vi "Init.vi"(8 "error in (no error)":errorcluster, 10 "Channel":i16, 11 "TrialBasedExperiment in":refnum<class "WNOriDiscExperiment.lvclass">) -> (0 "error out":errorcluster, 3 "TrialBasedExperiment out":refnum<class "WNOriDiscExperiment.lvclass">)   [LabVIEW 2014, in "WNOriDiscExperiment.lvclass"]
uses:
  WNOriDiscExperiment.lvclass
  TwoAfcEye/TwoAfcEye.lvclass
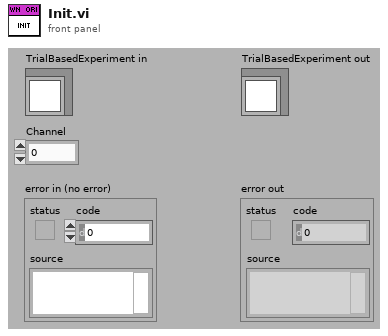
[diagram p1: front panel]
types:
  T1 = cluster{"Intertrial":dbl, "AcquireFixation":dbl, "HoldFixation":dbl, "DelayPeriod":dbl, "ResponsePeriod":dbl}
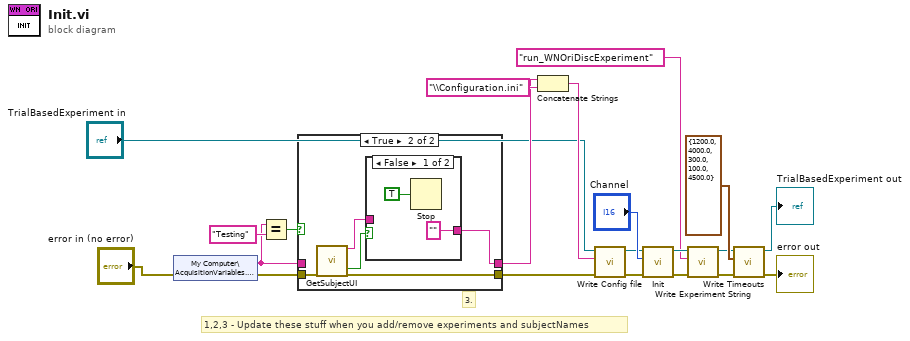
[diagram p0: block diagram]
diagram:
  # "1,2,3 - Update these stuff when you add/remove experiments and subjectNames"
  # "3."
  n1 = shared-variable "My Computer\\AcquisitionVariables.lvlib\\Subject"(error in="error in (no error)") -> (w17:string, error out=w16:errorcluster)
  n2 = Equal?(x=w17, y="Testing") -> (x = y?=w19:bool)
  n3 = case shown="True" w19 {
    tunnel: [w23 w28] -> w14
    tunnel: w17 -> [w23 _]
    tunnel: w16 -> [w22 w24]
    tunnel: [w22 w25] -> w15
    frame False {
    }
    frame True {
      n4 = call "GetSubjectUI.vi"("error in (no error)"=w24) -> ("subjectSelected"=w27:string, "OK"=w26:bool, "error out"=w25:errorcluster)  [unwired: 16 in]
      n5 = case shown="False" w26 {
        tunnel: w27 -> [_ w31]
        tunnel: ["" ("subjectSelected") w31] -> w28
        frame False {
          n6 = Stop(stop? (T)=TRUE) -> ()
        }
        frame True {
        }
      }
    }
  }
  n7 = Concatenate Strings(w14, "\\Configuration.ini") -> (w21:string)
  n8 = call-dynamic "Write Config file.vi"("error in (no error)"=w15, "Config file"=w21, "TrialBasedExperiment in"="TrialBasedExperiment in") -> ("error out"=w5:errorcluster, "TrialBasedExperiment out"=w6:refnum<class "WNOriDiscExperiment.lvclass">)  [unwired: 7 in]
  n9 = call-parent "Init.vi"("error in (no error)"=w5, "Channel"="Channel", "TrialBasedExperiment in"=w6) -> ("error out"=w4:errorcluster, "TrialBasedExperiment out"=w7:refnum<class "WNOriDiscExperiment.lvclass">)  [unwired: 7 in]
  n10 = call-dynamic "Write Experiment String.vi"("error in (no error)"=w4, "Experiment String"="run_WNOriDiscExperiment" ("string"), "TrialBasedExperiment in"=w7) -> ("error out"=w10:errorcluster, "TrialBasedExperiment out"=w9:refnum<class "WNOriDiscExperiment.lvclass">)  [unwired: 7 in]
  n11 = call-dynamic "Write Timeouts.vi"("error in (no error)"=w10, "Timeouts"=T1 {"Intertrial"=1200.0, "AcquireFixation"=4000.0, "HoldFixation"=300.0, "DelayPeriod"=100.0, "ResponsePeriod"=4500.0}, "TrialBasedExperiment in"=w9) -> ("error out"=→"error out":errorcluster, "TrialBasedExperiment out"=→"TrialBasedExperiment out":refnum<class "WNOriDiscExperiment.lvclass">)  [unwired: 7 in]
